vi "CameraSetModeAttr.vi"(8 "error in":errorcluster, 9 "Value":string="Manual", 10 "Attr String":string, 11 "IMAQdx Session In":T1) -> (0 "error out":errorcluster, 3 "IMAQdx Session out":T1)   [LabVIEW 2025]
doc: "Set the Mode of the attribute to Manual or Auto.\n\nThis software is licensed. Open the labview\\readme\\WPI Robotics Library Open Source License.txt file for more information."
uses:
  <vilib>/userDefined/High Color/IMAQdx.ctl
  <resource>/objmgr/imaqdx.rc
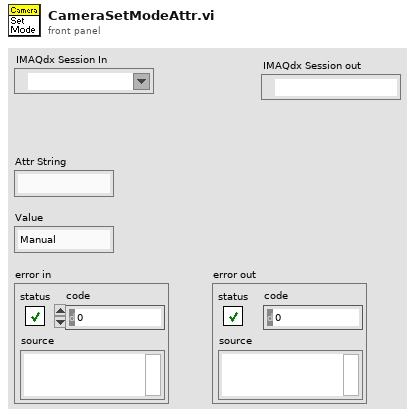
[diagram p1: front panel]
types:
  T1 = typedef "IMAQdx.ctl" = refnum<k21>
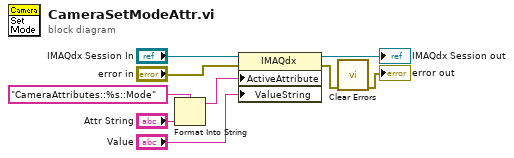
[diagram p0: block diagram]
diagram:
  n1 = Format Into String(format string="CameraAttributes::%s::Mode" ("Attr Format"), "Attr String") -> (resulting string=w1:string)  [unwired: 2 in, 1 out]
  n2 = property class="IMAQdx"(reference="IMAQdx Session In", error in="error in", "ActiveAttribute"=w1, "ValueString"="Value") -> (reference out=→"IMAQdx Session out":T1, error out=w6:errorcluster)
  n3 = call <vilib>:"Clear Errors.vi"("error in (no error)"=w6) -> ("error out"=→"error out":errorcluster)  [unwired: 5 in, 1 out]
